vi "rsp_New Connection.vi"(8 "error in":errorcluster, 9 "Data in":T1={"Connection Ref"=refnum, "Name"="", "Message Priority"=enum."Normal", "IP Address"=""}, 11 "DS TCP Listener in":refnum<class "DS TCP Listener.lvclass">) -> (0 "error out":errorcluster, 3 "dup DS TCP Listener out":refnum<class "DS TCP Listener.lvclass">)   [LabVIEW 2017, in "DS TCP Server.lvlib" / "DS TCP Listener.lvclass"]
doc: "This VI sends a <b>Public API Response</b> message to a registered MHL case of the Caller of the Worker that owns this VI.\n---"
uses:
  DS TCP Listener.lvclass
  C:/Program Files (x86)/National Instruments/LabVIEW 2017/vi.lib/addons/_Workers/Library/Classes/Worker/Worker.lvclass
  rsp_New Connection.ctl
  <vilib>/addons/_Workers/Library/Classes/Message/Priority.ctl
  DS TCP Listener.lvclass/DS TCP Listener.ctl
  <vilib>/addons/_Workers/Library/Classes/Worker/Worker.lvclass/Worker.ctl
  <vilib>/addons/_Workers/Library/Classes/Message/Enqueue Message to Queue.vi
  <vilib>/addons/_Workers/Library/Classes/Message/Message.lvclass
  <vilib>/addons/_Workers/Library/Classes/Worker/Worker.lvclass
  C:/Program Files (x86)/National Instruments/LabVIEW 2017/vi.lib/addons/_Workers/Library/Classes/Workers Object/Workers Object.lvclass
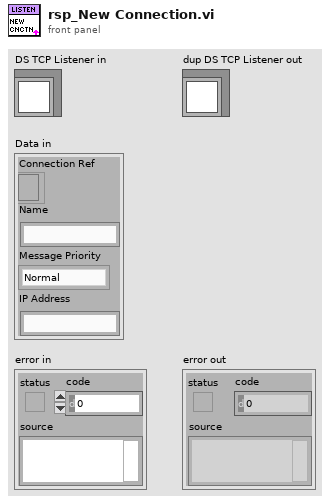
[diagram p1: front panel]
types:
  T1 = typedef "DS TCP Server.lvlib/DS TCP Listener.lvclass/rsp_New Connection.ctl" = cluster{"Connection Ref":refnum<k5>, "Name":string, "Message Priority":T2, "IP Address":string}
  T2 = typedef "Workers.lvlib/Message.lvclass/Priority.ctl" = enum16{"Low", "Normal", "High"}
  T3 = typedef "Workers.lvlib/Case Label.ctl" = string
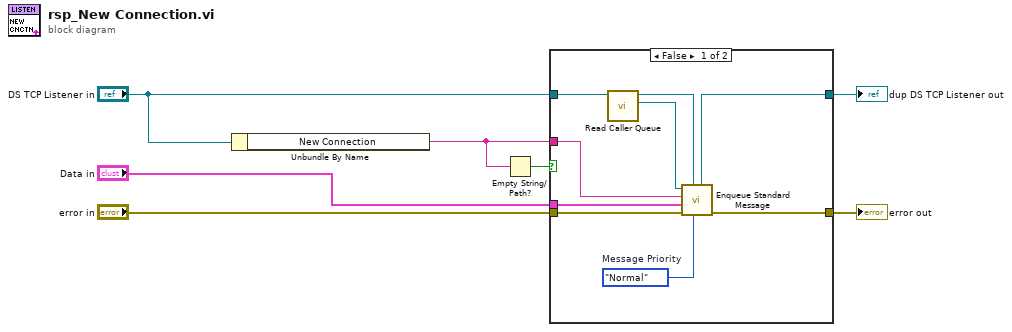
[diagram p0: block diagram]
diagram:
  n1 = Unbundle By Name("DS TCP Listener in") -> ("New Connection"=w2:T3)
  n2 = Empty String/Path?(string/path=w2) -> (empty?=w3:bool)
  n3 = case shown="False" w3 {
    tunnel: "error in" -> [w10 w17]
    tunnel: [w16 w17] -> w6
    tunnel: "Data in" -> [w14 _]
    tunnel: [w13 w18] -> w4
    tunnel: "DS TCP Listener in" -> [w11 w18]
    tunnel: w2 -> [w12 _]
    frame False {
      w15 = Priority."Normal"  # Message Priority
      n4 = call <vilib>:"Read Caller Queue.vi"("Worker_"=w11) -> ("Message Queue out"=w8:refnum<class "Message Queue.lvclass">, "dup Worker_out"=w9:refnum<class "DS TCP Listener.lvclass">)  [unwired: 9 in]
      n5 = call-poly <vilib>:"Enqueue Standard Message.vi"("Priority (Normal)"=w15, "Worker"=w9, "error in"=w10, "Data"=w14, "Case Label"=w12, "Message Queue"=w8) -> ("error out"=w16:errorcluster, "dup Worker out"=w13:refnum<class "DS TCP Listener.lvclass">)  [unwired: 3 in, 1 out]
    }
    frame True {
    }
  }
  "error out" <- w6
  "dup DS TCP Listener out" <- w4
